vi "mapTypeStringToProjectItemEnum.vi"(8 "error in (no error)":errorcluster, 10 "Type String":string, 11 "Project in":refnum<class "Project.lvclass">) -> (0 "error out":errorcluster, 2 "ProjectItemSelection":T1, 3 "Project out":refnum<class "Project.lvclass">)   [LabVIEW 2016, in "Project.lvclass"]
uses:
  Project.lvclass
  Typedefs/ProjectItemSelection.ctl
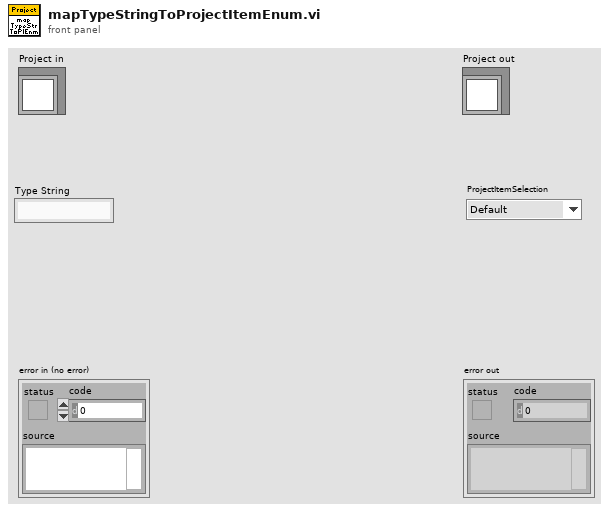
[diagram p1: front panel]
types:
  T1 = typedef "ProjectItemSelection.ctl" = enum16{"Default", "ClassPrivateData", "Dependencies", "Folder", "Library", "LVClass", "VI"}
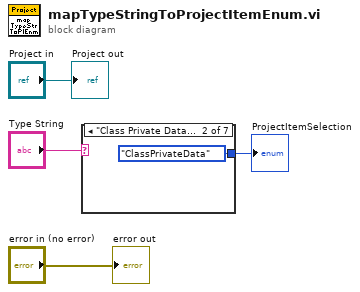
[diagram p0: block diagram]
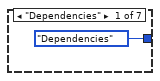
[diagram p2: hidden frame]
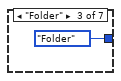
[diagram p3: hidden frame]
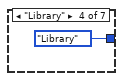
[diagram p4: hidden frame]
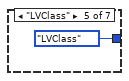
[diagram p5: hidden frame]
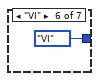
[diagram p6: hidden frame]
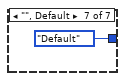
[diagram p7: hidden frame]
diagram:
  n1 = case shown="\"Class Private Data\"" "Type String" {
    tunnel: [ProjectItemSelection."Dependencies" ("ProjectItemSelection") ProjectItemSelection."ClassPrivateData" ("ProjectItemSelection") ProjectItemSelection."Folder" ("ProjectItemSelection") ProjectItemSelection."Library" ("ProjectItemSelection") ProjectItemSelection."LVClass" ("ProjectItemSelection") ProjectItemSelection."VI" ("ProjectItemSelection") ProjectItemSelection."Default" ("ProjectItemSelection")] -> w1
    frame "Dependencies" {
    }
    frame "Class Private Data" {
    }
    frame "Folder" {
    }
    frame "Library" {
    }
    frame "LVClass" {
    }
    frame "VI" {
    }
    frame "", Default {
    }
  }
  "ProjectItemSelection" <- w1
  "error out" <- "error in (no error)"
  "Project out" <- "Project in"
